vi "Error Query.vi"(8 "error in (no error)":errorcluster, 11 "VISA resource name":refnum<visa-resource-name>) -> (0 "error out":errorcluster, 1 "Error Message":string, 2 "Error Code":i32[](array[numeric]), 3 "VISA resource name out":refnum<visa-resource-name>)   [LabVIEW 2015, in "Keithley 2600 Series.lvlib"]
doc: "Queries the instrument for any errors in the instrument's error queue. It will continue to read errors until all errors have been read from the instrument. Any errors will be returned in the <B>error out</B> control.\n\n<B>Note:</B>\nThis VI is called automatically by most driver VIs so it is not usually necessary to call this in an application."
uses:
  Keithley 2600 Series.lvlib
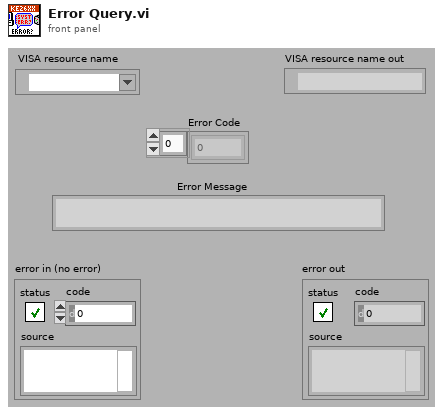
[diagram p1: front panel]
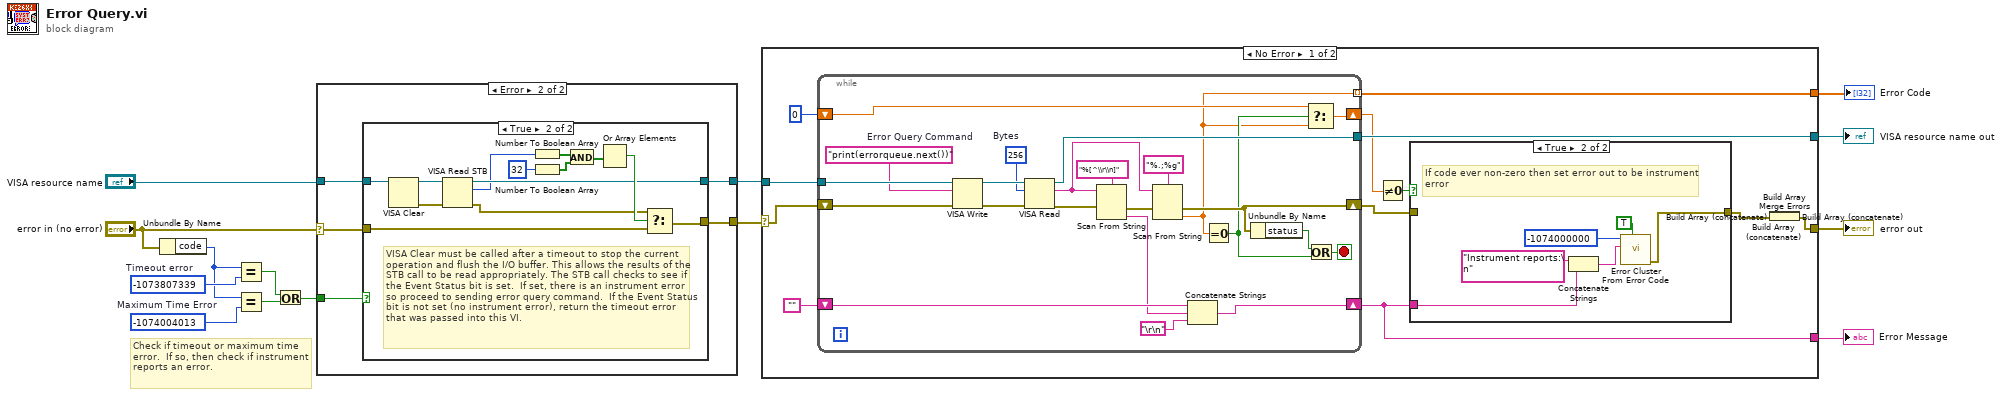
[diagram p0: block diagram]
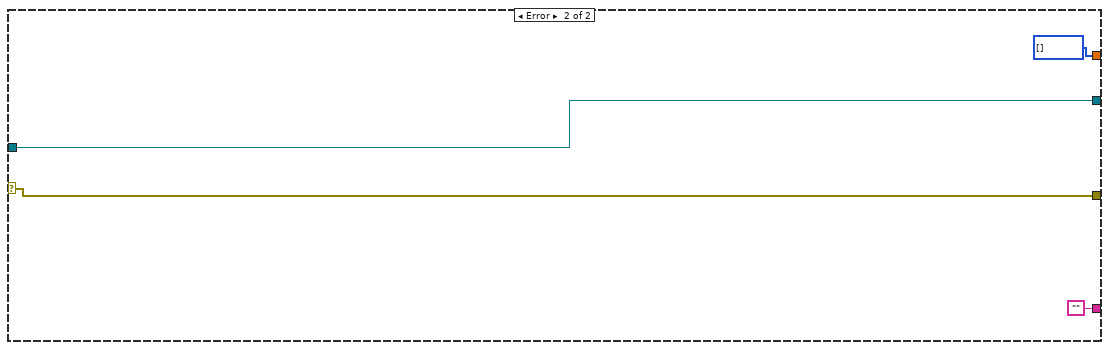
[diagram p5: hidden frame]
diagram:
  w5 = -1074004013  # Maximum Time Error
  w7 = -1073807339  # Timeout error
  # "Check if timeout or maximum time error.  If so, then check if instrument reports an error."
  n1 = Unbundle By Name("error in (no error)") -> ("code"=w6:i32)
  n2 = Equal?(x=w6, y=w7) -> (x = y?=w3:bool)
  n3 = Equal?(x=w6, y=w5) -> (x = y?=w4:bool)
  n4 = Or(x=w3, y=w4) -> (x .or. y?=w2:bool)
  n5 = case shown="Error" "error in (no error)" {
    selector: "error in (no error)" -> [w15 w19]
    tunnel: "VISA resource name" -> [w16 w21]
    tunnel: [w16 w20] -> w9
    tunnel: [w15 w18] -> w10
    tunnel: w2 -> [_ w17]
    frame No Error {
    }
    frame Error {
      n6 = case shown="True" w17 {
        tunnel: w21 -> [w23 w29]
        tunnel: [w23 w26] -> w20
        tunnel: w19 -> [w22 w32]
        tunnel: [w22 w31] -> w18
        frame False {
          # "Error code not a timeout, so best to pass on to user."
        }
        frame True {
          # "VISA Clear must be called after a timeout to stop the current operation and flush the I/O buffer. This allows the results of the  STB call to be read appropriately. The STB call checks to see if the Event Status bit is set.  If set, there is an instrument error so proceed to sending error query command.  If the Event Status bit is not set (no instrument error), return the timeout error that was passed into this VI."
          n7 = VISA Clear(VISA resource name=w29) -> (VISA resource name out=w28:refnum<visa-resource-name>, error out=w27:errorcluster)  [unwired: 1 in]
          n8 = VISA Read STB(8:w27, 11:w28) -> (0:w25:errorcluster, 2:w24:u16, 3:w26:refnum<visa-resource-name>)
          n9 = Number To Boolean Array(number=w24) -> (Boolean array=w33:bool[])
          n10 = Number To Boolean Array(number=32) -> (Boolean array=w35:bool[])
          n11 = And(x=w33, y=w35) -> (x .and. y?=w34:bool[])
          n12 = Or Array Elements(Boolean array=w34) -> (logical OR=w30:bool)
          n13 = Select(t=w25, s=w30, f=w32) -> (s? t:f=w31:errorcluster)
        }
      }
    }
  }
  n14 = case shown="No Error" w10 {
    selector: w10 -> [w41 w83]
    tunnel: [w52 w86] -> w14
    tunnel: w9 -> [w51 w86]
    tunnel: [w49 w83] -> w13
    tunnel: [w44 ""] -> w12
    tunnel: [w43 i32[] []] -> w11
    frame No Error {
      n15 = while {
        tunnel: [w82] -> w52
        tunnel: w51 -> [w81]
        shift-right: [w69] -> w44
        shift-left: "" -> [w72]
        shift-right: [w67] -> w45
        shift-left: 0 -> [w68]
        shift-right: [w65] -> w42
        shift-left: w41 -> [w66]
        tunnel: [w60] -> w43 mode=indexing
        stop <- w75 stop-if-true
        w79 = u32 256  # Bytes
        w77 = "print(errorqueue.next())"  # Error Query Command
        n16 = VISA Write(VISA resource name=w81, write buffer=w77, error in (no error)=w66) -> (VISA resource name out=w80:refnum<visa-resource-name>, error out=w78:errorcluster)  [unwired: 1 out]
        n17 = VISA Read(VISA resource name=w80, byte count=w79, error in (no error)=w78) -> (VISA resource name out=w82:refnum<visa-resource-name>, read buffer=w73:string, error out=w64:errorcluster)  [unwired: 1 out]
        n18 = Scan From String(format string="%[^\\r\\n]", input string=w73, error in=w64) -> (error out=w63:errorcluster, output 1=w70:string)  [unwired: 2 in, 2 out]
        n19 = Scan From String(format string="%.;%g", input string=w73, error in=w63) -> (error out=w65:errorcluster, output 1=w60:dbl)  [unwired: 2 in, 2 out]
        n20 = Concatenate Strings(w72, w70, "\r\n") -> (w69:string)
        n21 = Equal To 0?(x=w60) -> (x = 0?=w61:bool)
        n22 = Unbundle By Name(w65) -> ("status"=w62:bool)
        n23 = Select(t=w68, s=w61, f=w60) -> (s? t:f=w67:dbl)
        n24 = Or(x=w62, y=w61) -> (x .or. y?=w75:bool)
      }
      n25 = Not Equal To 0?(x=w45) -> (x != 0?=w47:bool)
      n26 = case shown="True" w47 {
        tunnel: w44 -> [_ w58]
        tunnel: [w53 w54] -> w46
        tunnel: w42 -> [w53 _]
        frame False {
        }
        frame True {
          # "If code ever non-zero then set error out to be instrument error"
          n27 = Concatenate Strings("Instrument reports:\n" ("Source"), w58) -> (w55:string)
          n28 = call <vilib>:"Error Cluster From Error Code.vi"("show call chain? (False)"=TRUE, "error message (\"\")"=w55, "error code (0)"=-1074000000 ("Code")) -> ("error out"=w54:errorcluster)  [unwired: 6 in]
        }
      }
      n29 = Build Array(w46) -> (w40:errorcluster[])
      n30 = Build Array (concatenate)(w40) -> (w39:errorcluster[])
      n31 = Build Array (concatenate)(w39) -> (w38:errorcluster[])
      n32 = Build Array (concatenate)(w38) -> (w37:errorcluster[])
      n33 = Merge Errors(w37) -> (w49:errorcluster)
    }
    frame Error {
    }
  }
  "VISA resource name out" <- w14
  "error out" <- w13
  "Error Message" <- w12
  "Error Code" <- w11
